vi "Vision Processing.vi"() -> ()   [LabVIEW 2011]
doc: "This VI runs in parallel to other tasks. It gets images from the camera, processes them for color or shape and use that information to affect robot behavior."
uses:
  <vilib>/Rock Robotics/WPI/Camera/WPI_CameraWhite Balance Values.ctl
  Robot Global Data.vi
  <vilib>/vision/NI_Vision_Development_Module.lvlib
panel:
  in  "lower limit":dbl=-0.05
  in  "upper limit":dbl=0.05
  out "Processed Image":T1(plugin-control)
  out "Original Image":T1(plugin-control)
  in  "Annotate":bool=TRUE
  in  "Particle Count Limit":i32=10
  in  "Area Size Limit":i32=444
  in  "Range":cluster{"Lower value":sgl, "Upper value":sgl}={"Lower value"=120.0, "Upper value"=255.0}
  out "X Position Array":dbl[](array[numeric])
  out "Y Position Array":dbl[](array[numeric])
  out "Number of Rectangles Visible":dbl
  in  "Turret Speed Limit":dbl=0.3
  out "Target 1":dbl[](array[numeric])
  out "Target 2":dbl[](array[numeric])
  out "Target 3":dbl[](array[numeric])
  out "Target 4":dbl[](array[numeric])
  out "Turret Rotation":dbl
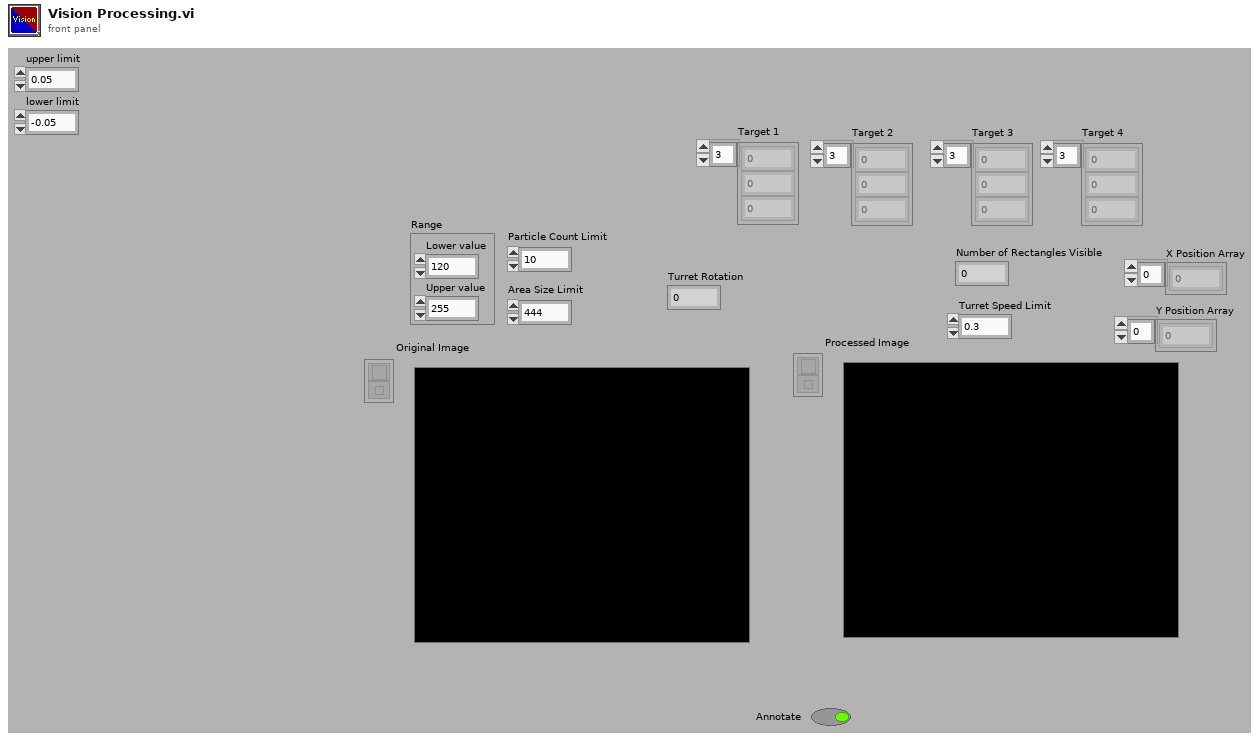
[diagram p1: front panel]
types:
  T1 = typedef "IMAQ Image.ctl" = refnum<image>
  T2 = typedef "WPI_CameraWhite Balance Values.ctl" = enum16{"Auto", "Fixed indoor", "Fixed outdoor 1", "Fixed outdoor 2", "Fixed fluorescent 1", "Fixed fluorescent 2", "Hold current"}
  T3 = typedef "Image Type" = u32
  T4 = typedef "WPI_CameraImageSize.ctl" = enum16{"640x480", "320x240", "160x120"}
  T5 = cluster{"fps":i32, "compression":i32, "Image Size":T4}
  T6 = typedef "WPI_CameraDevRef.ctl" = cluster{"Camera Address":string, "CameraStatus":errorcluster, "Acquire Image Notifier":refnum<notifier>}
  T7 = cluster{"Rect Coverage":dbl, "Aspect Ratio":dbl, "X Edge Strength":dbl, "Y Edge Strength":dbl}
  T8 = cluster{"Position":cluster{"X":dbl, "Y":dbl}, "Distance (ft)":dbl}[]
  T9 = cluster{cluster{"Left":dbl, "Top":dbl, "Right":dbl, "Bottom":dbl}, dbl[]}[]
  T10 = cluster{"Left":dbl, "Top":dbl, "Right":dbl, "Bottom":dbl}
  T11 = cluster{"Target Center (-1 to 1)":cluster{"X":dbl, "Y":dbl}, "Distance (ft)":dbl}
  T12 = cluster{"Target Center (-1 to 1)":cluster{"X":dbl, "Y":dbl}, "Distance (ft)":dbl}[]
  T13 = cluster{"Position":cluster{"X":dbl, "Y":dbl}, "Distance (ft)":dbl}
  T14 = cluster{"Axis 1":dbl, "Axis 2":dbl, "Axis 3":dbl, "Axis 4":dbl, "Axis 5":dbl, "Axis 6":dbl, "Button 1":bool, "Button 2":bool, "Button 3":bool, "Button 4":bool, "Button 5":bool, "Button 6":bool, "Button 7":bool, "Button 8":bool, "Button 9":bool, "Button 10":bool, "Button 11":bool, "Button 12":bool}
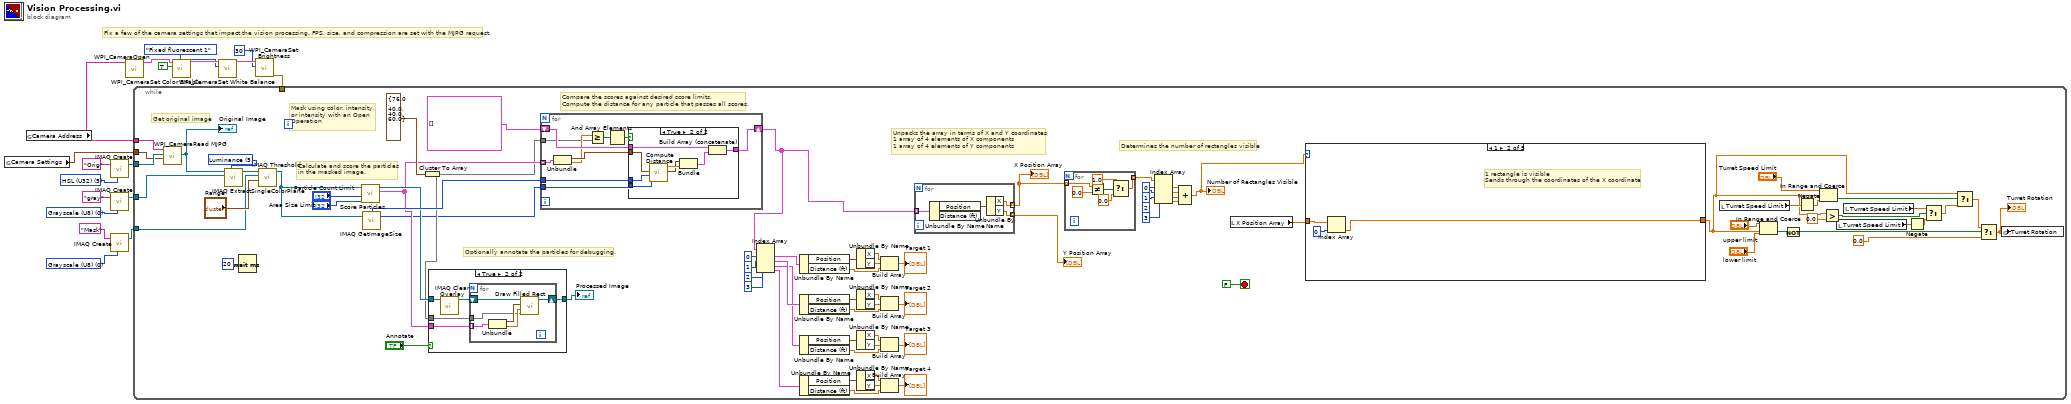
[diagram p0: block diagram]
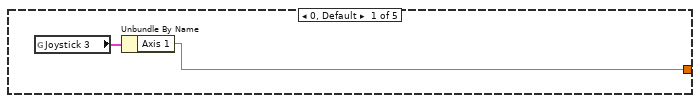
[diagram p2: hidden frame]
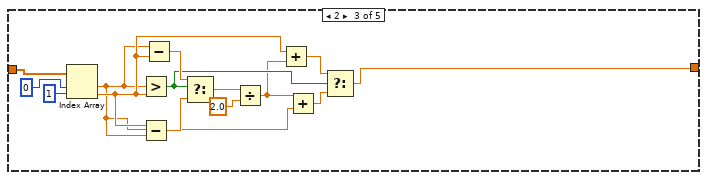
[diagram p3: hidden frame]
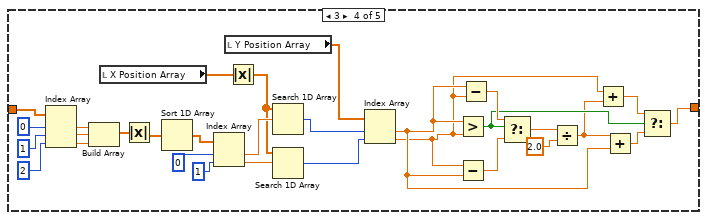
[diagram p4: hidden frame]
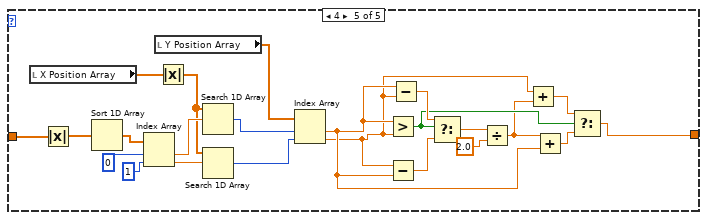
[diagram p5: hidden frame]
diagram:
  w11 = T3 0 items=["Grayscale (U8)", "Grayscale (I16)", "Grayscale (SGL)", "Complex (CSG)", "RGB (U32)", "HSL (U32)", "RGB (U64)", "Grayscale (U16)"] ("Image Type")
  w15 = T3 5 items=["Grayscale (U8)", "Grayscale (I16)", "Grayscale (SGL)", "Complex (CSG)", "RGB (U32)", "HSL (U32)", "RGB (U64)", "Grayscale (U16)"] ("Image Type")
  w18 = T3 0 items=["Grayscale (U8)", "Grayscale (I16)", "Grayscale (SGL)", "Complex (CSG)", "RGB (U32)", "HSL (U32)", "RGB (U64)", "Grayscale (U16)"] ("Image Type")
  # "Fix a few of the camera settings that impact the vision processing. FPS, size, and compression are set with the MJPG request."
  n1 = global read "Robot Global Data.vi" "Camera Settings"() -> (w1:T5)
  n2 = global read "Robot Global Data.vi" "Camera Address"() -> (w2:string)
  n3 = call "IMAQ Create"("Image Name"="Orig", "Image Type"=w15) -> ("New Image"=w14:T1)  [unwired: 2 in, 2 out]
  n4 = call "IMAQ Create"("Image Name"="gray", "Image Type"=w18) -> ("New Image"=w13:T1)  [unwired: 2 in, 2 out]
  n5 = call "IMAQ Create"("Image Name"="Mask", "Image Type"=w11) -> ("New Image"=w10:T1)  [unwired: 2 in, 2 out]
  n6 = call <vilib>:"WPI_CameraOpen.vi"("Camera Address"=w2) -> ("CameraDevRef"=w9:T6)  [unwired: 9 in, 1 out]
  n7 = call <vilib>:"WPI_CameraSet Color Enable.vi"("Color Enabled"=TRUE, "CameraDevRef"=w9) -> ("CameraDevRef Out"=w7:T6)  [unwired: 8 in, 1 out]
  n8 = call <vilib>:"WPI_CameraSet White Balance.vi"("White Balance"=WPI_CameraWhite_Balance_Values."Fixed fluorescent 1", "CameraDevRef"=w7) -> ("CameraDevRef Out"=w5:T6)  [unwired: 8 in, 1 out]
  n9 = call <vilib>:"WPI_CameraSet Brightness.vi"("Brightness"=30, "CameraDevRef"=w5) -> ("error out"=w3:errorcluster)  [unwired: 8 in, 1 out]
  n10 = while {
    tunnel: w14 -> [w100]
    tunnel: w13 -> [w82]
    tunnel: w10 -> [w84]
    tunnel: w2 -> [w99]
    tunnel: w3 -> [_]
    tunnel: w1 -> [w88]
    stop <- FALSE stop-if-true
    w87 = 5 items=["Red", "Green", "Blue", "Hue", "Saturation", "Luminance", "Value", "Intensity"] ("Color Plane")
    # "Determines the number of rectangles visible"
    # "Unpacks the array in terms of X and Y coordinates\n1 array of 4 elements of X components\n1 array of 4 elements of Y components"
    # "Optionally annotate the particles for debugging."
    # "Compare the scores against desired score limits.\nCompute the distance for any particle that passes all scores."
    # "Calculate and score the particles\nin the masked image."
    # "Mask using color, intensity,\nor intensity with an Open\nOperation"
    # "Get original image"
    n11 = call <vilib>:"WPI_CameraRead MJPG.vi"("Camera Settings"=w88, "Image"=w100, "address"=w99) -> ("Image Out"=w83:T1)  [unwired: 7 in, 1 out]
    "Original Image" <- w83
    n12 = call "IMAQ ExtractSingleColorPlane"("Color Plane"=w87, "Image Dst"=w82, "Image Src"=w83) -> ("Image Dst Out"=w85:T1)  [unwired: 1 in, 7 out]
    n13 = Wait (ms)(milliseconds to wait=u32 20) -> ()  [unwired: 1 out]
    n14 = call "IMAQ Threshold"("Range"="Range", "Image Dst"=w84, "Image Src"=w85) -> ("Image Dst Out"=w81:T1)  [unwired: 3 in, 5 out]
    n15 = call "Score Particles.vi"("Area Size Limit"="Area Size Limit", "Particle Count Limit"="Particle Count Limit", "Image Refnum in"=w81) -> ("Scored Particle Info"=w95:T9, "Image Refnum out"=w98:T1)  [unwired: 7 in]
    n16 = call "IMAQ GetImageSize"("Image"=w81) -> ("Y Resolution"=w89:i32, "X Resolution"=w101:i32)  [unwired: 3 in, 1 out]
    n17 = Cluster To Array(cluster=T7 {"Rect Coverage"=76.0, "Aspect Ratio"=40.0, "X Edge Strength"=40.0, "Y Edge Strength"=60.0} ("Score Limits")) -> (array=w93:dbl[])
    n18 = case shown="True" "Annotate" {
      tunnel: w98 -> [w184 w189]
      tunnel: [w184 w188] -> w96
      tunnel: w95 -> [_ w186]
      tunnel: w93 -> [_ w185]
      frame False {
      }
      frame True {
        n19 = call "IMAQ Clear Overlay"("Image"=w189) -> ("Image Out"=w187:T1)  [unwired: 2 in, 8 out]
        n20 = for {
          shift-right: [w194] -> w188
          shift-left: w187 -> [w195]
          tunnel: w186 -> [w191] mode=indexing
          tunnel: w185 -> [w190]
          n21 = Unbundle(w191) -> (w192:T10, w193:dbl[])
          n22 = call "Draw Filled Rect.vi"("Limits"=w190, "Scores"=w193, "Bounding Box"=w192, "image in"=w195) -> ("image out"=w194:T1)  [unwired: 7 in]
        }
      }
    }
    "Processed Image" <- w96
    n23 = for {
      shift-right: [w204] -> w57
      shift-left: T8 [] -> [w205]
      tunnel: w101 -> [w203]
      tunnel: w95 -> [w201] mode=indexing
      tunnel: w93 -> [w197]
      tunnel: w89 -> [w196]
      n24 = Unbundle(w201) -> (w202:T10, w198:dbl[])
      n25 = Greater Or Equal?(x=w198, y=w197) -> (x >= y?=w200:bool[])
      n26 = And Array Elements(Boolean array=w200) -> (logical AND=w199:bool)
      n27 = case shown="True" w199 {
        tunnel: w205 -> [w206 w214]
        tunnel: [w206 w213] -> w204
        tunnel: w202 -> [_ w209]
        tunnel: w203 -> [_ w211]
        tunnel: w196 -> [_ w207]
        frame False {
        }
        frame True {
          n28 = call "Compute Distance.vi"("Y Image Resolution"=w207, "X Image Resolution"=w211, "Bounding Box"=w209) -> ("Target Center (-1 to 1)"=w208:cluster{"X":dbl, "Y":dbl}, "Distance (ft)"=w210:dbl)  [unwired: 7 in]
          n29 = Bundle("Target Center (-1 to 1)"=w208, "Distance (ft)"=w210) -> (w212:T11)  [unwired: 1 in]
          n30 = Build Array (concatenate)(w214, w212) -> (w213:T12)
        }
      }
    }
    n31 = Index Array(array=w57, index #1=0 ("index"), index #2=1 ("index"), index #3=2 ("index"), index #4=3 ("index")) -> (element #1=w54:T13, element #2=w45:T13, element #3=w39:T13, element #4=w31:T13)
    n32 = Unbundle By Name(w54) -> ("Position"=w53:cluster{"X":dbl, "Y":dbl}, "Distance (ft)"=w50:dbl)
    n33 = Unbundle By Name(w45) -> ("Position"=w46:cluster{"X":dbl, "Y":dbl}, "Distance (ft)"=w48:dbl)
    n34 = Unbundle By Name(w39) -> ("Position"=w42:cluster{"X":dbl, "Y":dbl}, "Distance (ft)"=w40:dbl)
    n35 = Unbundle By Name(w31) -> ("Position"=w34:cluster{"X":dbl, "Y":dbl}, "Distance (ft)"=w36:dbl)
    n36 = Unbundle By Name(w53) -> ("X"=w52:dbl, "Y"=w51:dbl)
    n37 = Unbundle By Name(w46) -> ("X"=w44:dbl, "Y"=w47:dbl)
    n38 = Unbundle By Name(w42) -> ("X"=w38:dbl, "Y"=w41:dbl)
    n39 = Unbundle By Name(w34) -> ("X"=w32:dbl, "Y"=w35:dbl)
    n40 = Build Array(w52, w51, w50) -> (→"Target 1":dbl[])
    n41 = Build Array(w44, w47, w48) -> (→"Target 2":dbl[])
    n42 = Build Array(w38, w41, w40) -> (→"Target 3":dbl[])
    n43 = Build Array(w32, w35, w36) -> (→"Target 4":dbl[])
    n44 = for {
      tunnel: [w182] -> w55 mode=indexing
      tunnel: [w181] -> w73 mode=indexing
      tunnel: w57 -> [w180] mode=indexing
      n45 = Unbundle By Name(w180) -> ("Position"=w183:cluster{"X":dbl, "Y":dbl})  [unwired: 1 out]
      n46 = Unbundle By Name(w183) -> ("X"=w181:dbl, "Y"=w182:dbl)
    }
    "X Position Array" <- w73
    "Y Position Array" <- w55
    n47 = for {
      tunnel: w73 -> [w106] mode=indexing
      tunnel: [w102] -> w72 mode=indexing
      n48 = Not Equal?(x=w106, y=0.0) -> (x != y?=w105:bool)
      n49 = Select(t=1.0, s=w105, f=0.0) -> (s? t:f=w102:dbl)
    }
    n50 = Index Array(array=w72, index #1=0 ("index"), index #2=1 ("index"), index #3=2 ("index"), index #4=3 ("index")) -> (element #1=w70:dbl, element #2=w71:dbl, element #3=w69:dbl, element #4=w68:dbl)
    n51 = Compound Arithmetic op=ADD(w70, w71, w69, w68) -> (w62:dbl)
    "Number of Rectangles Visible" <- w62
    n52 = local read "X Position Array"() -> (w79:dbl[])
    n53 = case shown="1" w62 {
      tunnel: w79 -> [_ w112 w126 w156 w159]
      tunnel: [w108 w110 w113 w128 w158] -> w26
      frame 0, Default {
        n54 = global read "Robot Global Data.vi" "Joystick 3"() -> (w109:T14)
        n55 = Unbundle By Name(w109) -> ("Axis 1"=w108:dbl)
      }
      frame 1 {
        # "1 rectangle is visible\nSends through the coordinates of the X coordinate"
        n56 = Index Array(array=w112, index=0) -> (element=w110:dbl)
      }
      frame 2 {
        n57 = Index Array(array=w126, index #1=0 ("index"), index #2=1 ("index")) -> (element #1=w114:dbl, element #2=w115:dbl)
        n58 = Greater?(x=w114, y=w115) -> (0:w119:bool)
        n59 = Subtract(x=w115, y=w114) -> (x-y=w122:dbl)
        n60 = Subtract(x=w114, y=w115) -> (x-y=w123:dbl)
        n61 = Select(t=w123, s=w119, f=w122) -> (s? t:f=w121:dbl)
        n62 = Divide(x=w121, y=2.0) -> (x/y=w116:dbl)
        n63 = Add(x=w115, y=w116) -> (x+y=w118:dbl)
        n64 = Add(x=w116, y=w114) -> (x+y=w117:dbl)
        n65 = Select(t=w118, s=w119, f=w117) -> (s? t:f=w113:dbl)
      }
      frame 3 {
        n66 = Index Array(array=w156, index #1=0 ("index"), index #2=1 ("index"), index #3=2 ("index")) -> (element #1=w152:dbl, element #2=w151:dbl, element #3=w150:dbl)
        n67 = Build Array(w152, w151, w150) -> (w149:dbl[])
        n68 = local read "X Position Array"() -> (w142:dbl[])
        n69 = Absolute Value(x=w149) -> (abs(x)=w148:dbl[])
        n70 = Sort 1D Array(array=w148) -> (sorted array=w147:dbl[])
        n71 = Index Array(array=w147, index #1=0 ("index"), index #2=1 ("index")) -> (element #1=w144:dbl, element #2=w143:dbl)
        n72 = local read "Y Position Array"() -> (w140:dbl[])
        n73 = Absolute Value(x=w142) -> (abs(x)=w127:dbl[])
        n74 = Search 1D Array(1D array=w127, element=w144) -> (index of element=w141:i32)  [unwired: 1 in]
        n75 = Search 1D Array(1D array=w127, element=w143) -> (index of element=w139:i32)  [unwired: 1 in]
        n76 = Index Array(array=w140, index #1=w141, index #2=w139) -> (element #1=w130:dbl, element #2=w129:dbl)
        n77 = Greater?(x=w130, y=w129) -> (0:w134:bool)
        n78 = Subtract(x=w129, y=w130) -> (x-y=w137:dbl)
        n79 = Subtract(x=w130, y=w129) -> (x-y=w138:dbl)
        n80 = Select(t=w138, s=w134, f=w137) -> (s? t:f=w136:dbl)
        n81 = Divide(x=w136, y=2.0) -> (x/y=w131:dbl)
        n82 = Add(x=w129, y=w131) -> (x+y=w133:dbl)
        n83 = Add(x=w131, y=w130) -> (x+y=w132:dbl)
        n84 = Select(t=w133, s=w134, f=w132) -> (s? t:f=w128:dbl)
      }
      frame 4 {
        n85 = local read "X Position Array"() -> (w173:dbl[])
        n86 = Absolute Value(x=w159) -> (abs(x)=w179:dbl[])
        n87 = Sort 1D Array(array=w179) -> (sorted array=w178:dbl[])
        n88 = Index Array(array=w178, index #1=0 ("index"), index #2=1 ("index")) -> (element #1=w175:dbl, element #2=w174:dbl)
        n89 = local read "Y Position Array"() -> (w171:dbl[])
        n90 = Absolute Value(x=w173) -> (abs(x)=w157:dbl[])
        n91 = Search 1D Array(1D array=w157, element=w175) -> (index of element=w172:i32)  [unwired: 1 in]
        n92 = Search 1D Array(1D array=w157, element=w174) -> (index of element=w170:i32)  [unwired: 1 in]
        n93 = Index Array(array=w171, index #1=w172, index #2=w170) -> (element #1=w161:dbl, element #2=w160:dbl)
        n94 = Greater?(x=w161, y=w160) -> (0:w165:bool)
        n95 = Subtract(x=w160, y=w161) -> (x-y=w168:dbl)
        n96 = Subtract(x=w161, y=w160) -> (x-y=w169:dbl)
        n97 = Select(t=w169, s=w165, f=w168) -> (s? t:f=w167:dbl)
        n98 = Divide(x=w167, y=2.0) -> (x/y=w162:dbl)
        n99 = Add(x=w160, y=w162) -> (x+y=w164:dbl)
        n100 = Add(x=w162, y=w161) -> (x+y=w163:dbl)
        n101 = Select(t=w164, s=w165, f=w163) -> (s? t:f=w158:dbl)
      }
    }
    n102 = local read "Turret Speed Limit"() -> (w29:dbl)
    n103 = In Range and Coerce(upper limit="upper limit", x=w26, lower limit="lower limit") -> (In Range?=w76:bool)  [unwired: 1 out]
    n104 = Not(x=w76) -> (.not. x?=w77:bool)
    n105 = Negate(x=w29) -> (-x=w28:dbl)
    n106 = In Range and Coerce(upper limit="Turret Speed Limit", x=w26, lower limit=w28) -> (In Range?=w27:bool)  [unwired: 1 out]
    n107 = Greater?(x=w26, y=0.0) -> (0:w23:bool)
    n108 = local read "Turret Speed Limit"() -> (w21:dbl)
    n109 = local read "Turret Speed Limit"() -> (w22:dbl)
    n110 = Negate(x=w21) -> (-x=w20:dbl)
    n111 = Select(t=w22, s=w23, f=w20) -> (s? t:f=w19:dbl)
    n112 = Select(t=w26, s=w27, f=w19) -> (s? t:f=w24:dbl)
    n113 = Select(t=w24, s=w77, f=0.0) -> (s? t:f=w56:dbl)
    "Turret Rotation" <- w56
    n114 = global write "Robot Global Data.vi" "Turret Rotation"(w56) -> ()
  }
